vi "report.vi"() -> ()   [LabVIEW 2017]
uses:
  <vilib>/addons/database/Connection.llb/DB Tools Open Connec (Path).vi
  <vilib>/Utility/file.llb/Write Delimited Spreadsheet (string).vi
  <vilib>/addons/database/NI_Database_API.lvlib
panel:
  in  "delete":bool
  in  "Scan Barcode":bool
  out "error out":errorcluster
  in  "error in (no error)":errorcluster
  in  "FROM":timestamp format="%<%x>T"
  in  "TO":timestamp format="%<%x>T"
  out "table":string[][](table)
  out "Table header":string[](array[string])
  in  "Barcode":string
  in  "Type Wise":enum16{"Barcode Wise", "Datewise"}(ring)=enum."Datewise"
  in  "stop":bool
  in  "Export to Excel":bool
  in  "Get Report":bool
  # "Data History"
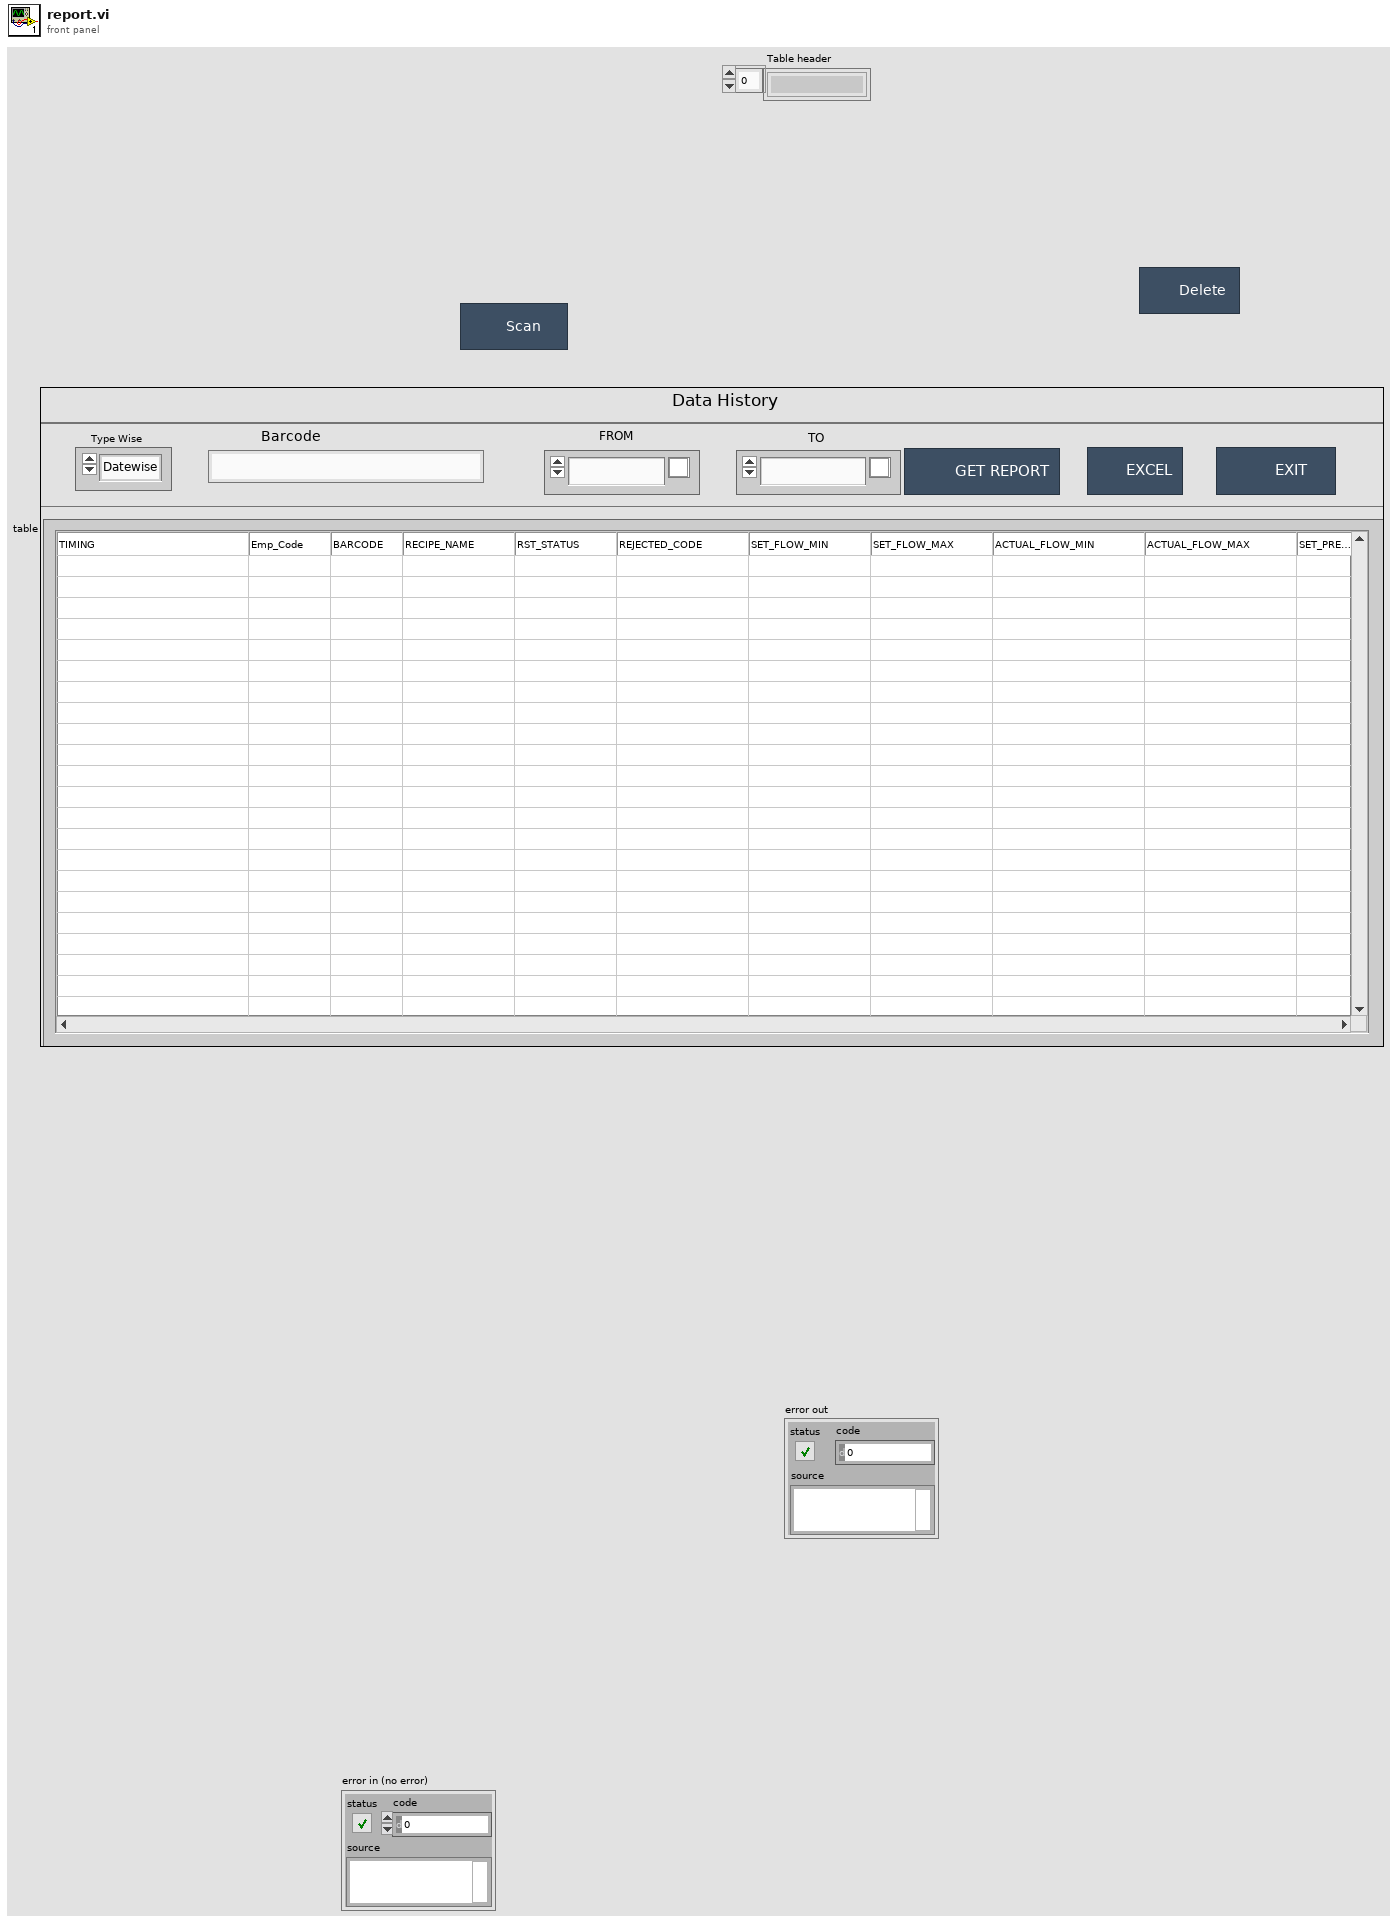
[diagram p1: front panel]
types:
  T1 = typedef "LVDateTimeRec.ctl" = cluster{"fractional second":dbl, "second":i32, "minute":i32, "hour":i32, "day of month":i32, "month":i32, "year":i32, "day of week":i32, "day of year":i32, "DST":i32}
  T2 = typedef "NI_Database_API.lvlib/Conn ObjectReference.ctl" = refnum<k1>
  T3 = enum32{"invalid app kind", "Development System", "Run Time System", "Student Edition", "Embedded LabVIEW", "Evaluation", "Custom"}
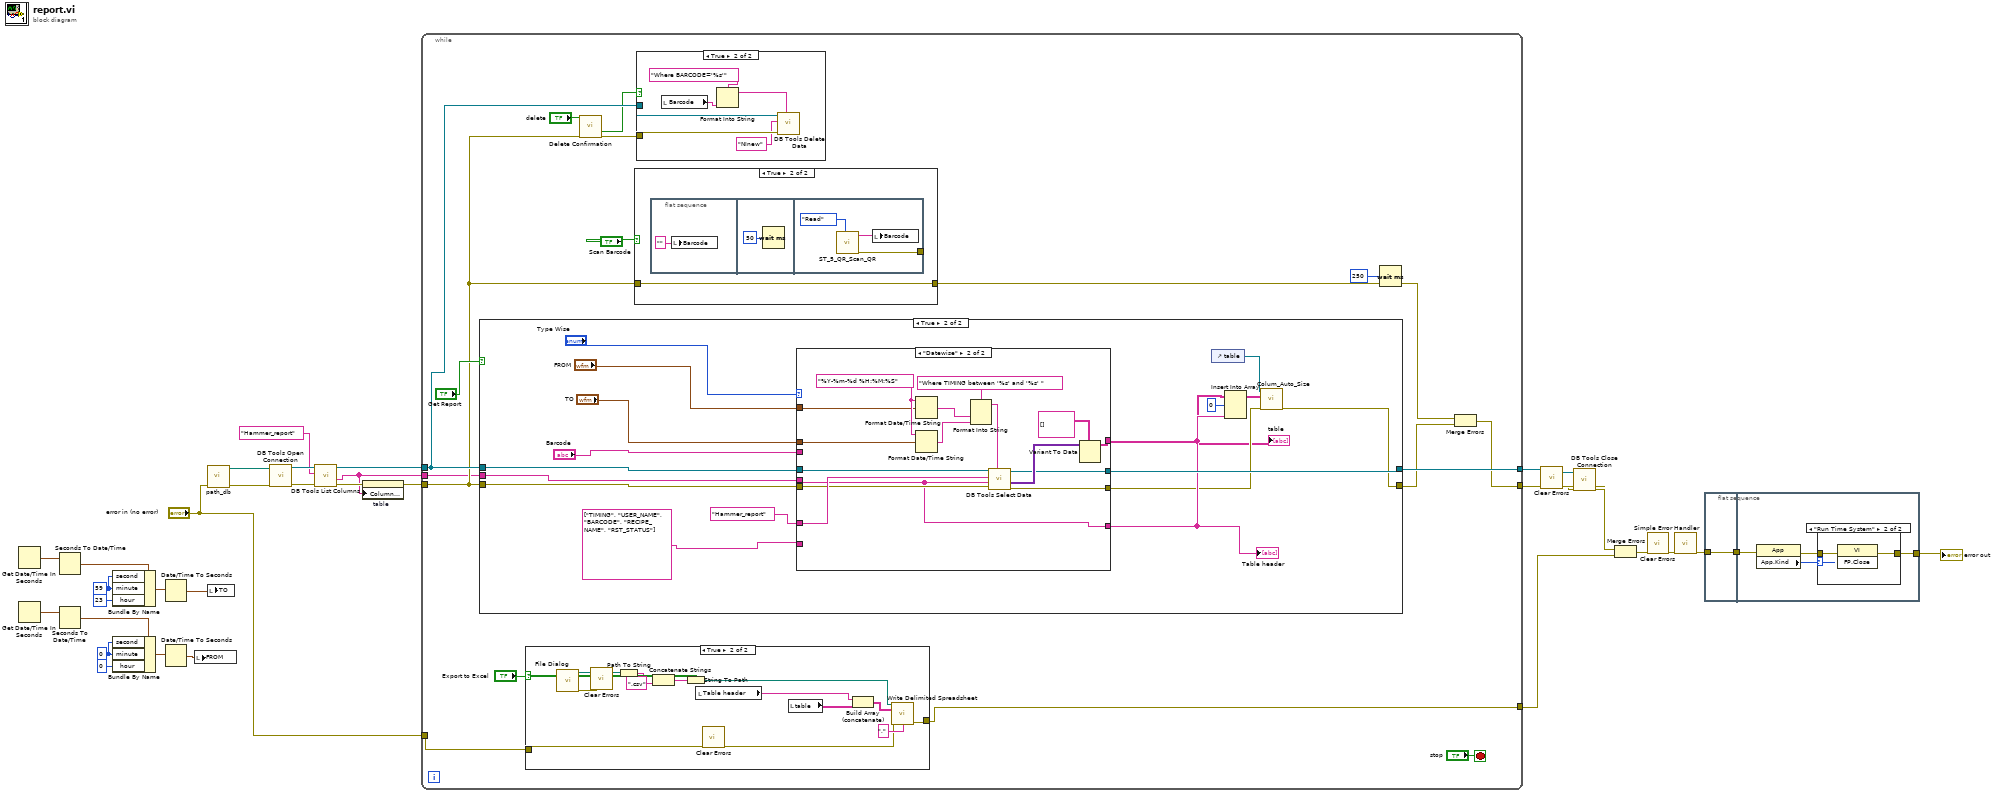
[diagram p0: block diagram]
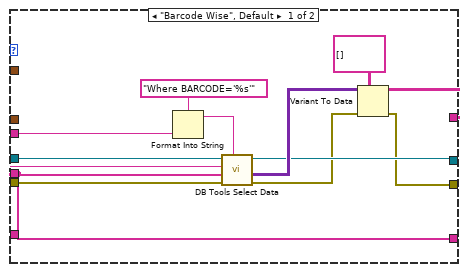
[diagram p7: hidden frame]
diagram:
  w26 = 0 ("minute")
  w27 = 59 ("minute")
  n1 = Get Date/Time In Seconds() -> (seconds since 1Jan1904=w29:timestamp)
  n2 = Get Date/Time In Seconds() -> (seconds since 1Jan1904=w24:timestamp)
  n3 = Seconds To Date/Time(time stamp (now)=w29) -> (date time rec=w30:T1)  [unwired: 1 in]
  n4 = Seconds To Date/Time(time stamp (now)=w24) -> (date time rec=w23:T1)  [unwired: 1 in]
  n5 = Bundle By Name(cluster=w30, "second"=w27, "minute"=w27, "hour"=23) -> (w31:T1)
  n6 = Bundle By Name(cluster=w23, "second"=w26, "minute"=w26, "hour"=0) -> (w22:T1)
  n7 = Date/Time To Seconds(2:w31) -> (0:w20:timestamp)  [unwired: 1 in]
  n8 = Date/Time To Seconds(2:w22) -> (0:w21:timestamp)  [unwired: 1 in]
  n9 = local write "FROM"(w21) -> ()
  n10 = call "path_db.vi"("error in"="error in (no error)") -> ("error out"=w11:errorcluster, "resulting string"=w12:path)  [unwired: 9 in]
  n11 = local write "TO"(w20) -> ()
  n12 = call-poly <vilib>:"DB Tools Open Connection.vi"("error in (no error)"=w11, "connection information"=w12) -> ("error out"=w7:errorcluster, "connection reference"=w6:T2)  [unwired: 6 in]
  n13 = call <vilib>:"DB Tools List Columns.vi"("error in (no error)"=w7, "table"="Hammer_report", "connection reference"=w6) -> ("error out"=w3:errorcluster, "columns"=w1:string[], "connection reference out"=w5:T2)  [unwired: 1 in, 1 out]
  n14 = property on="table" class="Tbl (strict)"(error in=w3, "Column Headers[]"=w1) -> (error out=w2:errorcluster)  [unwired: 1 in, 1 out]
  n15 = while {
    tunnel: w5 -> [w38]
    tunnel: w2 -> [w37]
    tunnel: [w49] -> w19
    tunnel: [w39] -> w9
    tunnel: "error in (no error)" -> [w47]
    tunnel: [w46] -> w17
    tunnel: w1 -> [w33]
    stop <- "stop" stop-if-true
    n16 = case shown="True" "Get Report" {
      tunnel: w38 -> [w78 w94]
      tunnel: w37 -> [w77 w93]
      tunnel: [w78 w92] -> w49
      tunnel: [w77 w86] -> w40
      tunnel: w33 -> [_ w79]
      frame False {
      }
      frame True {
        n17 = case shown="\"Datewise\"" "Type Wise" {
          tunnel: w94 -> [w108 w124]
          tunnel: w93 -> [w107 w110]
          tunnel: string[] ["TIMING", "USER_NAME", "BARCODE", "RECIPE_NAME", "RST_STATUS"] -> [_ _]
          tunnel: "Hammer_report" ("table") -> [w102 w121]
          tunnel: [w101 w120] -> w92
          tunnel: [w99 w119] -> w82
          tunnel: [w98 w113] -> w80
          tunnel: [w96 w109] -> w88
          tunnel: "Barcode" -> [w97 _]
          tunnel: "FROM" -> [_ w112]
          tunnel: "TO" -> [_ w111]
          tunnel: w79 -> [w96 w109]
          frame "Barcode Wise", Default {
            n18 = Format Into String(format string="Where BARCODE='%s'", w97) -> (resulting string=w105:string)  [unwired: 2 in, 1 out]
            n19 = call <vilib>:"DB Tools Select Data.vi"("condition"=w105, "error in (no error)"=w107, "columns"=w96, "table"=w102, "connection reference"=w108) -> ("error out"=w100:errorcluster, "data"=w104:variant[][], "connection reference out"=w101:T2)  [unwired: 1 in]
            n20 = Variant To Data(error in=w100, type=string[][] [], Variant=w104) -> (data=w98:string[][], error out=w99:errorcluster)
          }
          frame "Datewise" {
            w115 = "%Y-%m-%d %H:%M:%S" ("time format string (%c)")
            n21 = Format Date/Time String(time format string (%c)=w115, seconds (now)=w111) -> (date/time string=w116:string)  [unwired: 1 in]
            n22 = Format Date/Time String(time format string (%c)=w115, seconds (now)=w112) -> (date/time string=w117:string)  [unwired: 1 in]
            n23 = Format Into String(format string="Where TIMING between '%s' and '%s' ", w117, w116) -> (resulting string=w118:string)  [unwired: 2 in, 1 out]
            n24 = call <vilib>:"DB Tools Select Data.vi"("condition"=w118, "error in (no error)"=w110, "columns"=w109, "table"=w121, "connection reference"=w124) -> ("error out"=w119:errorcluster, "data"=w123:variant[][], "connection reference out"=w120:T2)  [unwired: 1 in]
            n25 = Variant To Data(type=string[][] [], Variant=w123) -> (data=w113:string[][])  [unwired: 1 in, 1 out]
          }
        }
        "table" <- w80
        "Table header" <- w88
        n26 = control-ref of="table"() -> (w85:refnum<vi>)
        n27 = Insert Into Array(array=w80, index (row)=0, new element=w88) -> (w84:string[][])  [unwired: 1 in]
        n28 = call "Colum_Auto_Size.vi"("error in (no error)"=w82, "Table With header"=w84, "Table reference"=w85) -> ("error out"=w86:errorcluster)  [unwired: 8 in]
      }
    }
    n29 = case shown="True" "Export to Excel" {
      tunnel: w47 -> [w63 w76]
      tunnel: [w63 w75] -> w46
      frame False {
      }
      frame True {
        n30 = call "File Dialog"() -> ("selected path"=w69:path, "error out"=w70:errorcluster)  [unwired: 12 in, 2 out]
        n31 = call <vilib>:"Clear Errors.vi"("error in (no error)"=w70) -> ()  [unwired: 5 in, 2 out]
        n32 = Path To String(path=w69) -> (string=w68:string)
        n33 = Concatenate Strings(w68, ".csv" ("string")) -> (w66:string)
        n34 = String To Path(string=w66) -> (path=w65:path)
        n35 = local read "Table header"() -> (w72:string[])
        n36 = call <vilib>:"Clear Errors.vi"("error in (no error)"=w76) -> ("error out"=w64:errorcluster)  [unwired: 5 in, 1 out]
        n37 = local read "table"() -> (w73:string[][])
        n38 = Build Array (concatenate)(w72, w73) -> (w74:string[][])
        n39 = call-poly <vilib>:"Write Delimited Spreadsheet.vi"("file path (dialog if empty)"=w65, "2D data"=w74, "error in (no error)"=w64, "delimiter (\\t)"="," ("delimiter (\\t)")) -> ("error out"=w75:errorcluster)  [unwired: 10 in, 1 out]
      }
    }
    n40 = call "Delete Confirmation"("Enable"="delete", "error in (no error)"=w37) -> ("OK"=w34:bool, "error out"=w36:errorcluster)  [unwired: 16 in]
    n41 = case shown="True" "Scan Barcode" {
      tunnel: w37 -> [w56 w57]
      tunnel: [w56 w57] -> w41
      frame False {
      }
      frame True {
        n42 = flat-sequence {
          tunnel: [w60] -> _
          frame #0 {
            n43 = local write "Barcode"("" ("Barcode")) -> ()
          }
          frame #1 {
            n44 = Wait (ms)(milliseconds to wait=u32 50) -> ()  [unwired: 1 out]
          }
          frame #2 {
            n45 = call "ST_5_QR_Scan_QR.vi"("Enum"=enum16{"Read", "Write"}."Read") -> ("error out"=w60:errorcluster, "LB QR ST 5"=w62:string)  [unwired: 9 in]
            n46 = local write "Barcode"(w62) -> ()
          }
        }
      }
    }
    n47 = case shown="True" w34 {
      tunnel: w38 -> [_ w55]
      tunnel: w36 -> [_ w54]
      frame False {
      }
      frame True {
        n48 = local read "Barcode"() -> (w53:string)
        n49 = Format Into String(format string="Where BARCODE='%s'", w53) -> (resulting string=w52:string)  [unwired: 2 in, 1 out]
        n50 = call <vilib>:"DB Tools Delete Data.vi"("condition"=w52, "error in (no error)"=w54, "table"="NInew", "connection reference"=w55) -> ()  [unwired: 6 in, 2 out]
      }
    }
    n51 = Wait (ms)(milliseconds to wait=u32 250) -> ()  [unwired: 1 out]
    n52 = Merge Errors(w41, w40) -> (w39:errorcluster)
  }
  n53 = call <vilib>:"Clear Errors.vi"("error in (no error)"=w9) -> ("error out"=w8:errorcluster)  [unwired: 5 in, 1 out]
  n54 = call <vilib>:"DB Tools Close Connection.vi"("error in (no error)"=w8, "connection reference"=w19) -> ("error out"=w18:errorcluster)  [unwired: 5 in]
  n55 = Merge Errors(w18, w17) -> (w16:errorcluster)
  n56 = call <vilib>:"Clear Errors.vi"("error in (no error)"=w16) -> ("error out"=w15:errorcluster)  [unwired: 5 in, 1 out]
  n57 = call <vilib>:"Simple Error Handler.vi"("error in (no error)"=w15) -> ("error out"=w14:errorcluster)  [unwired: 4 in, 4 out]
  n58 = flat-sequence {
    tunnel: w14 -> [w125]
    tunnel: [w125] -> w32
    tunnel: w32 -> [w127]
    tunnel: [w126] -> w13
    frame #0 {
    }
    frame #1 {
      n59 = property class="App"(error in=w127) -> (error out=w128:errorcluster, "App.Kind"=w129:T3)  [unwired: 1 in, 1 out]
      n60 = case shown="\"Run Time System\"" w129 {
        tunnel: w128 -> [w130 w132]
        tunnel: [w130 w131] -> w126
        frame Default {
        }
        frame "Run Time System" {
          n61 = invoke class="VI" method="FP.Close"(error in=w132) -> (error out=w131:errorcluster)  [unwired: 2 in, 2 out]
        }
      }
    }
  }
  "error out" <- w13
